vi "ZE_Recorder_OrderChannels.vi"(8 "error in":errorcluster, 11 "Channel Array In":T1 caption="Channel Array" {"Terminal" items=["Default"=-1, "RSE"=10083, "NRSE"=10078, "Differential"=10106, "Pseudodifferential"=12529]}) -> (0 "error out":errorcluster, 2 "channels rearranged":bool, 3 "Channel Array Out":T1 caption="Channel Array" {"Terminal" items=["Default"=-1, "RSE"=10083, "NRSE"=10078, "Differential"=10106, "Pseudodifferential"=12529]})   [LabVIEW 2025, in "ZE_Recorder.lvlib"]
doc: "ZE_Recorder_OrderChannels.vi\n----------------------------------------------\nThis VI rearanges the channels per device and by channel name as assignment of channels to tasks can only be done on sorted channels.\n\nInputs:\n---------------------\n- error in : Cluster; \n- Channel Array : 1DArrayOfCluster; \n\nOutputs:\n---------------------\n- error out : Cluster; \n- channels rearranged : Boolean; \n- Channel Array : 1DArrayOfCluster; \n\n----------------------------------------------\n25.12.2016\nZühlke Engineering AG\nCH-8952 Schlieren\nwww.zuehlke.com"
uses:
  ZE_Recorder.lvlib
  ZE_Recorder_ChannelCluster.ctl
  ChannelCluster.ctl
  ZE_Recorder_Units.ctl
  Temperature.ctl
panel:
  # "Connector Pane"
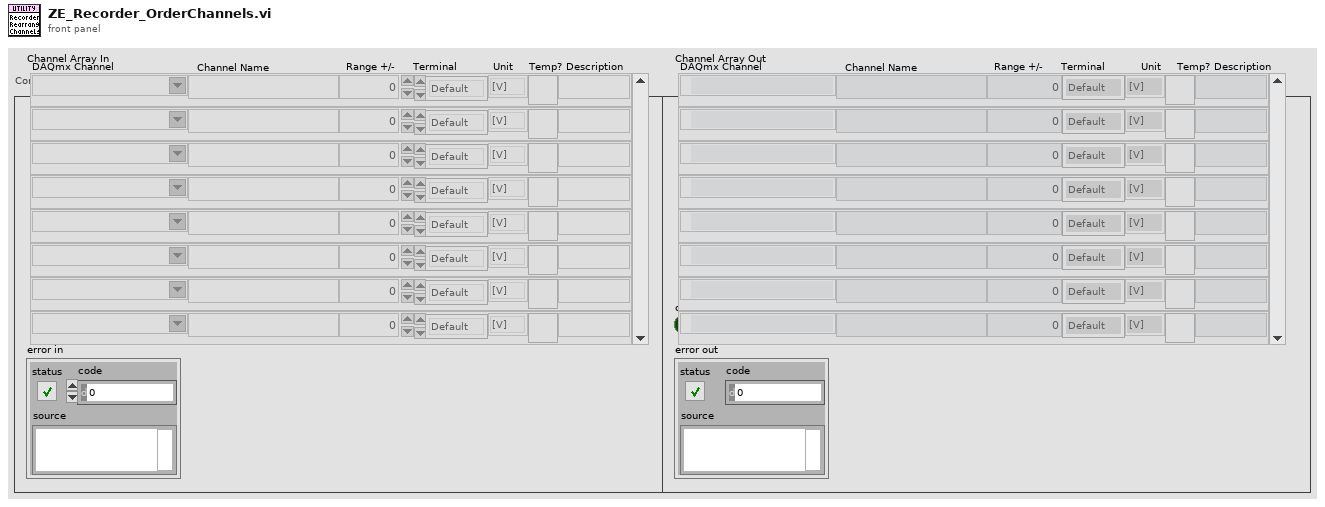
[diagram p1: front panel]
types:
  T1 = typedef "ZE_Recorder.lvlib/ZE_Recorder_ChannelCluster.ctl" = T2[]
  T2 = typedef "ZE_Recorder.lvlib/ChannelCluster.ctl" = cluster{"physical channel":tag, "channel name":string, "Range":dbl, "Terminal":i32, "Unit":T3, "isTemp":T4, "Description":string}
  T3 = typedef "ZE_Recorder.lvlib/ZE_Recorder_Units.ctl" = enum16{"[V]", "[A]", "[F]", "[H]", "[°C]", "[ml/s]", "[m/s]", "[bar]", "[%]", "[N]", "[?]"}
  T4 = typedef "ZE_Recorder.lvlib/Temperature.ctl" = bool
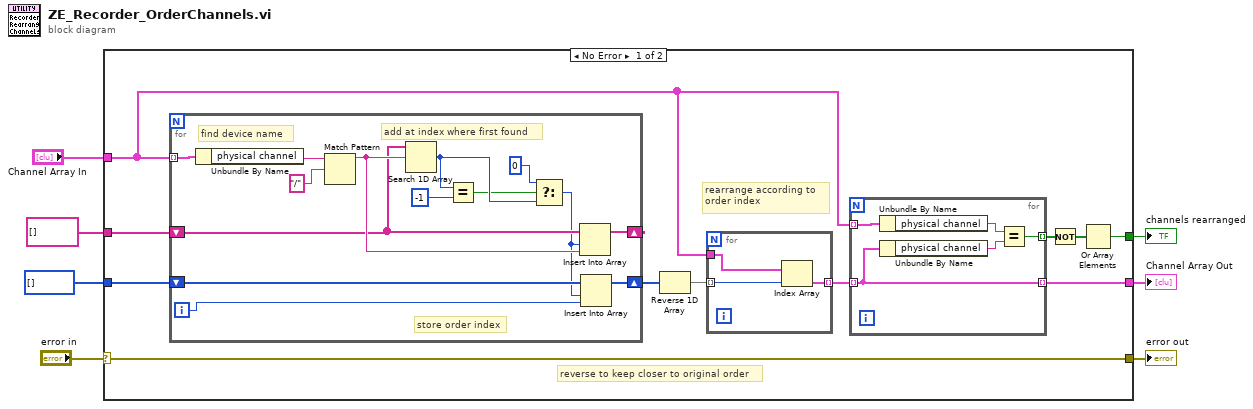
[diagram p0: block diagram]
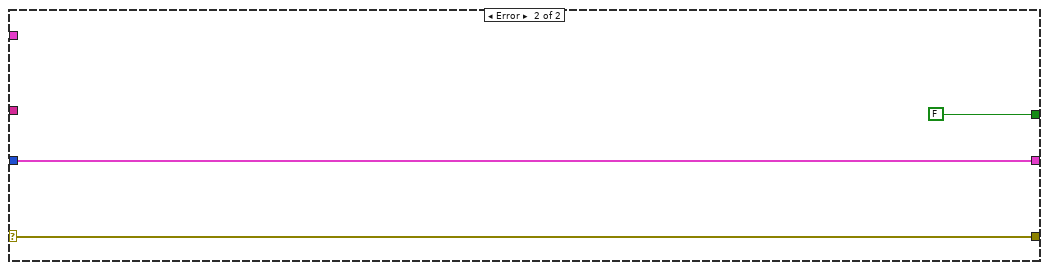
[diagram p2: hidden frame]
diagram:
  n1 = case shown="No Error" "error in" {
    selector: "error in" -> [w10 w41]
    tunnel: string[] [] -> [w18 _]
    tunnel: i32[] [] -> [w17 _]
    tunnel: "Channel Array In" -> [w13 w43]
    tunnel: [w12 w43] -> w1
    tunnel: [w11 FALSE] -> w4
    tunnel: [w10 w41] -> w3
    frame No Error {
      # "rearrange according to \norder index"
      # "reverse to keep closer to original order"
      n2 = for {
        tunnel: w13 -> [w40] mode=indexing
        shift-right: [w32] -> w16
        shift-left: w17 -> [w34]
        shift-right: [w33] -> _
        shift-left: w18 -> [w36]
        i -> [w35]
        # "store order index"
        # "add at index where first found"
        # "find device name"
        n3 = Unbundle By Name(w40) -> ("physical channel"=w39:tag)
        n4 = Match Pattern(string=w39, regular expression="/") -> (before substring=w37:string)  [unwired: 1 in, 3 out]
        n5 = Search 1D Array(1D array=w36, element=w37) -> (index of element=w28:i32)  [unwired: 1 in]
        n6 = Equal?(x=w28, y=-1) -> (x = y?=w27:bool)
        n7 = Select(t=0, s=w27, f=w28) -> (s? t:f=w31:i32)
        n8 = Insert Into Array(array=w36, index=w31, new element=w37) -> (w33:string[])
        n9 = Insert Into Array(array=w34, index=w31, new element=w35) -> (w32:i32[])
      }
      n10 = Reverse 1D Array(array=w16) -> (reversed array=w15:i32[])
      n11 = for {
        tunnel: w15 -> [w26] mode=indexing
        tunnel: [w25] -> w14 mode=indexing
        tunnel: w13 -> [w24]
        n12 = Index Array(array=w24, index=w26) -> (element=w25:T2)
      }
      n13 = for {
        tunnel: w14 -> [w22] mode=indexing
        tunnel: w13 -> [w23] mode=indexing
        tunnel: [w22] -> w12 mode=indexing
        tunnel: [w19] -> w9 mode=indexing
        n14 = Unbundle By Name(w23) -> ("physical channel"=w21:tag)
        n15 = Unbundle By Name(w22) -> ("physical channel"=w20:tag)
        n16 = Equal?(x=w21, y=w20) -> (x = y?=w19:bool)
      }
      n17 = Not(x=w9) -> (.not. x?=w8:bool[])
      n18 = Or Array Elements(Boolean array=w8) -> (logical OR=w11:bool)
    }
    frame Error {
    }
  }
  "channels rearranged" <- w4
  "error out" <- w3
  "Channel Array Out" <- w1
